vi "Periodic Tasks.vi"(8 "error in":errorcluster) -> ()   [LabVIEW 2018]
doc: "This VI runs in parallel to other tasks. It can contain as many user-defined periodic loops as you need. These can carry out PID or other sorts of timed response."
uses:
  <vilib>/Rock Robotics/WPI/Solenoid/WPI_SolenoidValue.ctl
  <vilib>/Rock Robotics/WPI/Utilities/WPI_GetSetVariantRefNum.vi
  <vilib>/Rock Robotics/WPI/Ultrasonic/WPI_SonarSRF04DigitalRefNum Registry Get.vi
  <vilib>/Rock Robotics/Network Tables/NT Read Boolean.vi
  <vilib>/Rock Robotics/Network Tables/NT Write Boolean.vi
  <vilib>/Rock Robotics/Network Tables/NT Write Number.vi
  <vilib>/Rock Robotics/WPI/Solenoid/Deprecated/WPI_SolenoidSetBool.vi
  <vilib>/Rock Robotics/WPI/Solenoid/WPI_SolenoidSetEnum.vi
  <vilib>/Rock Robotics/WPI/Ultrasonic/WPI_SonarSRF04DigitalGetRange.vi
panel:
  out "Encoder_Val":dbl
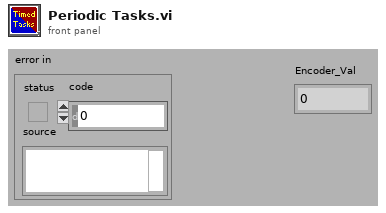
[diagram p1: front panel]
types:
  T1 = typedef "WPI_JoystickDevRef.ctl" = cluster{"Device":T2}
  T2 = typedef "WPI_JoystickDeviceEnum.ctl" = enum16{"USB 0", "USB 1", "USB 2", "USB 3", "USB 4", "USB 5"}
  T3 = typedef "WPI_RobotDriveDevRef.ctl" = cluster{"DevStatus":errorcluster, "Motors[]":T4[], "Square Inputs":bool, "Max Output":dbl}
  T4 = typedef "WPI_MotorControlDeviceRef.ctl" = cluster{"DeviceStatus":errorcluster, "Type":T5, "PWM":cluster{"PWM Channel":T6, "DeadBand":T7}, "CAN":cluster{"Device Number":u8, "SetOutput VI Ref":variant, "GetOutput VI Ref":variant, "Enable VI Ref":variant, "Disable VI Ref":variant, "Data":variant}, "Invert":bool, "DIO PWM":cluster{"PWM \"Enable\" Channel":T6, "DIOChannel":T8, "PWM Rate":dbl}}
  T5 = typedef "WPI_MotorControlType.ctl" = enum16{"PWM", "CAN", "DIO PWM"}
  T6 = typedef "FPGA_DIOPWMChannel.ctl" = enum8{"PWM 0", "PWM 1", "PWM 2", "PWM 3", "PWM 4", "PWM 5", "PWM 6", "PWM 7", "PWM 8", "PWM 9", "PWM MXP 0", "PWM MXP 1", "PWM MXP 2", "PWM MXP 3", "PWM MXP 4", "PWM MXP 5", "PWM MXP 6", "PWM MXP 7", "PWM MXP 8", "PWM MXP 9", "Invalid"}
  T7 = typedef "WPI_PWMDeadband.ctl" = cluster{"Name":string, "maxPositivePwm":i32, "minPositivePwm":i32, "centerPwm":i32, "maxNegativePwm":i32, "minNegativePwm":i32, "angularRange":u16}
  T8 = typedef "FPGA_DIOChannel.ctl" = enum8{"DIO 0", "DIO 1", "DIO 2", "DIO 3", "DIO 4", "DIO 5", "DIO 6", "DIO 7", "DIO 8", "DIO 9", "DIO MXP 0", "DIO MXP 1", "DIO MXP 2", "DIO MXP 3", "DIO MXP 4", "DIO MXP 5", "DIO MXP 6", "DIO MXP 7", "DIO MXP 8", "DIO MXP 9", "DIO MXP 10", "DIO MXP 11", "DIO MXP 12", "DIO MXP 13", "DIO MXP 14", "DIO MXP 15", "SPI Port CS1", "SPI Port CS2", "SPI Port CS3", "SPI Port MISO", "SPI Port MOSI", "Invalid"}
  T9 = typedef "WPI_SolenoidDevRef.ctl" = cluster{"DevStatus":errorcluster, "Pneumatics Control Module":u8, "Forward Solenoid Channel":T10, "Reverse Solenoid Channel":T10}
  T10 = typedef "WPI_SolenoidChannel.ctl" = enum8{"Solenoid 0", "Solenoid 1", "Solenoid 2", "Solenoid 3", "Solenoid 4", "Solenoid 5", "Solenoid 6", "Solenoid 7", "Invalid"}
  T11 = typedef "WPI_UltrasonicDeviceRef.ctl" = cluster{"DevStatus":errorcluster, "Ping Channel":T8, "Echo Channel":T8, "CntIndex":T12}
  T12 = typedef "FPGA_CounterCtrSystemIndex.ctl" = enum8{"Ctr 0", "Ctr 1", "Ctr 2", "Ctr 3", "Ctr 4", "Ctr 5", "Ctr 6", "Ctr 7", "Invalid"}
  T13 = typedef "WPI_SwitchDevRef.ctl" = cluster{"DevStatus":errorcluster, "DIO Channel":T8, "CntIndex":T12, "Normally Closed":bool}
  T14 = typedef "WPI_EncoderDevRef.ctl" = cluster{"DevStatus":errorcluster, "EncoderIndex":T15, "CounterIndex":T12, "DistancePerCount":dbl, "Decoding Type":T16}
  T15 = typedef "FPGA_EncoderIdx.ctl" = enum8{"Enc 0", "Enc 1", "Enc 2", "Enc 3", "Enc 4", "Enc 5", "Enc 6", "Enc 7", "Invalid"}
  T16 = typedef "WPI_EncoderType.ctl" = enum16{"1x", "2x", "4x"}
  T17 = cluster{"JoystickDevRef":T1, "RobotDriveDevRef":T3}
  T18 = typedef "WPI_CompressorDevRef.ctl" = cluster{"DevStatus":errorcluster, "Pneumatics Control Module":u8}
  T19 = typedef "WPI_SolenoidValue.ctl" = enum16{"Off", "On", "Forward", "Reverse"}
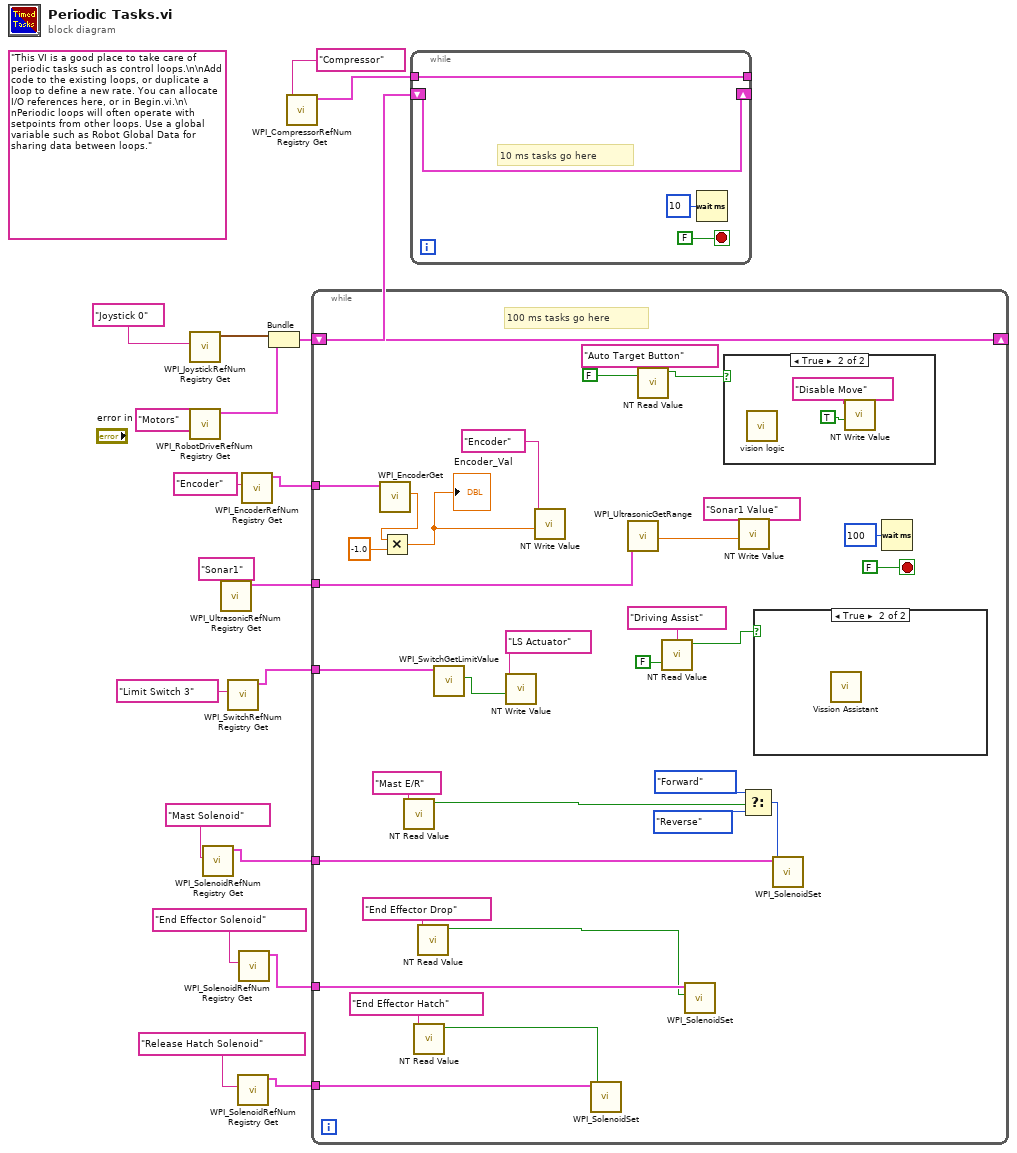
[diagram p0: block diagram]
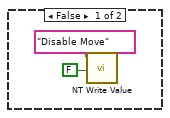
[diagram p3: hidden frame]
diagram:
  (unwired) "This VI is a good place to take care of periodic tasks such as control loops.\n\nAdd code to the existing loops, or duplicate a loop to define a new rate. You can allocate I/O references here, or in Begin.vi.\n\nPeriodic loops will often operate with setpoints from other loops. Use a global variable such as Robot Global Data for sharing data between loops."
  n1 = call <vilib>:"WPI_JoystickRefNum Registry Get.vi"("refnum name"="Joystick 0") -> ("JoystickDevRef"=w17:T1)  [unwired: 1 in, 9 out]
  n2 = call <vilib>:"WPI_RobotDriveRefNum Registry Get.vi"("refnum name"="Motors") -> ("RobotDriveDevRef"=w16:T3)  [unwired: 1 in, 9 out]
  n3 = call <vilib>:"WPI_SolenoidRefNum Registry Get.vi"("refnum name"="Mast Solenoid") -> ("SolenoidDevRef"=w8:T9)  [unwired: 9 in, 1 out]
  n4 = call-poly <vilib>:"WPI_UltrasonicRefNum Registry Get.vi"("refnum name"="Sonar1") -> ("SonarSRF04DevRef"=w13:T11)  [unwired: 9 in, 1 out]
  n5 = call <vilib>:"WPI_SwitchRefNum Registry Get.vi"("refnum name"="Limit Switch 3") -> ("SwitchDevRef"=w11:T13)  [unwired: 9 in, 1 out]
  n6 = call <vilib>:"WPI_SolenoidRefNum Registry Get.vi"("refnum name"="Release Hatch Solenoid") -> ("SolenoidDevRef"=w3:T9)  [unwired: 9 in, 1 out]
  n7 = call <vilib>:"WPI_SolenoidRefNum Registry Get.vi"("refnum name"="End Effector Solenoid") -> ("SolenoidDevRef"=w5:T9)  [unwired: 9 in, 1 out]
  n8 = call <vilib>:"WPI_EncoderRefNum Registry Get.vi"("refnum name"="Encoder") -> ("EncoderDevRef"=w1:T14)  [unwired: 9 in, 1 out]
  n9 = Bundle("JoystickDevRef"=w17, "RobotDriveDevRef"=w16) -> (w15:T17)  [unwired: 1 out]
  n10 = call <vilib>:"WPI_CompressorRefNum Registry Get.vi"("refnum name"="Compressor") -> ("CompressorDevRef"=w9:T18)  [unwired: 9 in, 1 out]
  n11 = while {
    shift-right: [w49] -> _
    shift-left: w15 -> [w49]
    tunnel: w13 -> [w48]
    tunnel: w11 -> [w42]
    tunnel: w8 -> [w27]
    tunnel: w5 -> [w32]
    tunnel: w3 -> [w31]
    tunnel: w1 -> [w24]
    stop <- FALSE stop-if-true
    # "100 ms tasks go here"
    n12 = call <vilib>:"WPI_EncoderGet.vi"("EncoderDevRef"=w24) -> ("Distance"=w21:dbl)  [unwired: 5 in, 5 out]
    n13 = Multiply(x=w21, y=-1.0) -> (x*y=w22:dbl)
    "Encoder_Val" <- w22
    n14 = call-poly <vilib>:"NT Read Value.vi"("Name"="Mast E/R") -> ("Boolean"=w26:bool)  [unwired: 9 in, 1 out]
    n15 = call-poly <vilib>:"NT Read Value.vi"("Name"="End Effector Hatch") -> ("Boolean"=w33:bool)  [unwired: 9 in, 1 out]
    n16 = call-poly <vilib>:"NT Read Value.vi"("Name"="End Effector Drop") -> ("Boolean"=w25:bool)  [unwired: 9 in, 1 out]
    n17 = call <vilib>:"WPI_SwitchGetLimitValue.vi"("SwitchDevRef"=w42) -> ("Switch Pressed"=w41:bool)  [unwired: 8 in, 2 out]
    n18 = call-poly <vilib>:"NT Write Value.vi"("Boolean"=w41, "Name"="LS Actuator") -> ()  [unwired: 9 in, 1 out]
    n19 = call-poly <vilib>:"NT Write Value.vi"("Numeric"=w22, "Name"="Encoder") -> ()  [unwired: 9 in, 1 out]
    n20 = call-poly <vilib>:"WPI_SolenoidSet.vi"("Value"=w33, "SolenoidDevRef"=w31) -> ()  [unwired: 8 in, 2 out]
    n21 = call-poly <vilib>:"WPI_UltrasonicGetRange.vi"("SonarSRF04DevRef"=w48) -> ("Distance"=w47:dbl)  [unwired: 8 in, 2 out]
    n22 = call-poly <vilib>:"NT Read Value.vi"("Default Value"=FALSE, "Name"="Auto Target Button") -> ("Boolean"=w44:bool)  [unwired: 8 in, 1 out]
    n23 = call-poly <vilib>:"NT Read Value.vi"("Default Value"=FALSE, "Name"="Driving Assist") -> ("Boolean"=w37:bool)  [unwired: 8 in, 1 out]
    n24 = call-poly <vilib>:"WPI_SolenoidSet.vi"("Value"=w25, "SolenoidDevRef"=w32) -> ()  [unwired: 8 in, 2 out]
    n25 = case shown="True" w44 {
      frame False {
        n26 = call-poly <vilib>:"NT Write Value.vi"("Boolean"=FALSE, "Name"="Disable Move") -> ()  [unwired: 9 in, 1 out]
      }
      frame True {
        n27 = call "vision logic.vi"() -> ()  [unwired: 16 in]
        n28 = call-poly <vilib>:"NT Write Value.vi"("Boolean"=TRUE, "Name"="Disable Move") -> ()  [unwired: 9 in, 1 out]
      }
    }
    n29 = call-poly <vilib>:"NT Write Value.vi"("Numeric"=w47, "Name"="Sonar1 Value") -> ()  [unwired: 9 in, 1 out]
    n30 = Select(t=WPI_SolenoidValue."Forward" ("Value"), s=w26, f=WPI_SolenoidValue."Reverse" ("Value")) -> (s? t:f=w28:T19)
    n31 = case shown="True" w37 {
      frame False {
      }
      frame True {
        n32 = call "Vission Assistant.vi"() -> ()  [unwired: 12 in]
      }
    }
    n33 = call-poly <vilib>:"WPI_SolenoidSet.vi"("Value"=w28, "SolenoidDevRef"=w27) -> ()  [unwired: 8 in, 2 out]
    n34 = Wait (ms)(milliseconds to wait=u32 100) -> ()  [unwired: 1 out]
  }
  n35 = while {
    shift-right: [w57] -> _
    shift-left: w15 -> [w57]
    tunnel: w9 -> [w56]
    tunnel: [w56] -> _
    stop <- FALSE stop-if-true
    # "10 ms tasks go here"
    n36 = Wait (ms)(milliseconds to wait=u32 10) -> ()  [unwired: 1 out]
  }
